vi "PicoScopeospaOpen.vi"(5 "Serial Number":string, 7 "Use Serial Number":bool, 8 "error in (no error)":errorcluster, 9 "Mode":u16(ring) items=["Dialog On Error", "no dialog - CloseUnit and Stop", "no dialog - Continue", "no dialog - Stop"], 10 "Resolution":u32(ring) items=["8-bit"=0, "12-bit"=1, "14-bit"=2, "15-bit"=3, "16-bit"=4, "10-bit"=10]) -> (0 "error out":errorcluster, 1 "Max ADC value":i16, 2 "Device Info":T2, 3 "handle out":i16, 4 "psospa Units":string, 6 "serialLth":i16)   [LabVIEW 2010]
doc: "This VI manages listing and opens devices with device details."
uses:
  psospa.dll
panel:
  out "PICO_USB_POWER_DETAILS":T1 {"dataPort_"."currentRdo_" format="%x"; "powerport_"."currentPdo_" format="%x"; "powerport_"."currentRdo_" format="%x"}
  out "minValue":i16
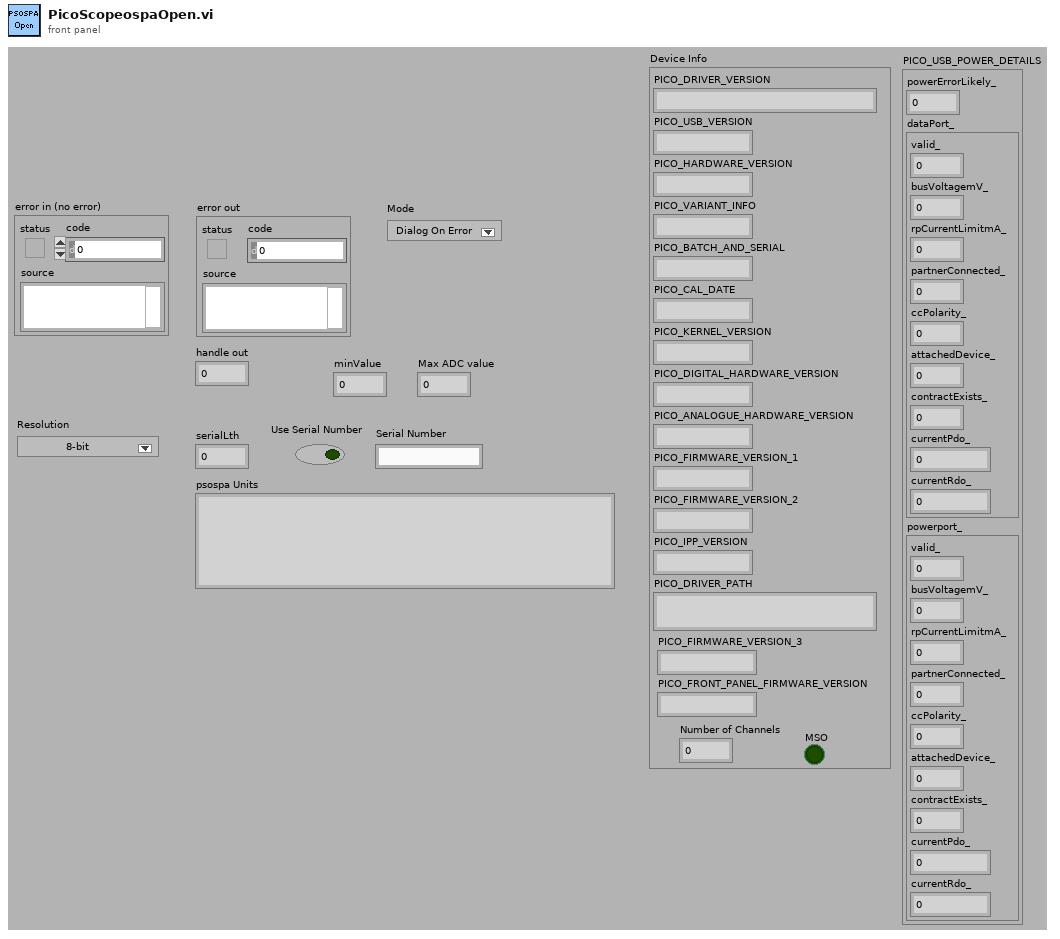
[diagram p1: front panel]
types:
  T1 = cluster{"powerErrorLikely_":u8, "dataPort_":cluster{"valid_":u8, "busVoltagemV_":u32, "rpCurrentLimitmA_":u32, "partnerConnected_":u8, "ccPolarity_":u8, "attachedDevice_":u32, "contractExists_":u8, "currentPdo_":u32, "currentRdo_":u32}, "powerport_":cluster{"valid_":u8, "busVoltagemV_":u32, "rpCurrentLimitmA_":u32, "partnerConnected_":u8, "ccPolarity_":u8, "attachedDevice_":u32, "contractExists_":u8, "currentPdo_":u32, "currentRdo_":u32}}
  T2 = cluster{"PICO_DRIVER_VERSION":string, "PICO_USB_VERSION":string, "PICO_HARDWARE_VERSION":string, "PICO_VARIANT_INFO":string, "PICO_BATCH_AND_SERIAL":string, "PICO_CAL_DATE":string, "PICO_KERNEL_VERSION":string, "PICO_DIGITAL_HARDWARE_VERSION":string, "PICO_ANALOGUE_HARDWARE_VERSION":string, "PICO_FIRMWARE_VERSION_1":string, "PICO_FIRMWARE_VERSION_2":string, "PICO_IPP_VERSION":string, "PICO_DRIVER_PATH":string, "PICO_FIRMWARE_VERSION_3":string, "PICO_FRONT_PANEL_FIRMWARE_VERSION":string, "Number of Channels":i16, "MSO":bool}
  T3 = cluster{"status":bool, "code":u32, "source":string}
  T4 = cluster{"PICO_DRIVER_VERSION":string, "PICO_USB_VERSION":string, "PICO_HARDWARE_VERSION":string, "PICO_VARIANT_INFO":string, "PICO_BATCH_AND_SERIAL":string, "PICO_CAL_DATE":string, "PICO_KERNEL_VERSION":string, "PICO_DIGITAL_HARDWARE_VERSION":string, "PICO_ANALOGUE_HARDWARE_VERSION":string, "PICO_FIRMWARE_VERSION_1":string, "PICO_FIRMWARE_VERSION_2":string, "PICO_IPP_VERSION":string, "PICO_DRIVER_PATH":string, "PICO_FIRMWARE_VERSION_3":string, "PICO_FRONT_PANEL_FIRMWARE_VERSION":string}
  T5 = cluster{"PICO_DRIVER_VERSION":string, "PICO_USB_VERSION":string, "PICO_HARDWARE_VERSION":string, "PICO_VARIANT_INFO":string, "PICO_BATCH_AND_SERIAL":string, "PICO_CAL_DATE":string, "PICO_KERNEL_VERSION":string, "PICO_DIGITAL_HARDWARE_VERSION":string, "PICO_ANALOGUE_HARDWARE_VERSION":string, "PICO_FIRMWARE_VERSION_1":string, "PICO_FIRMWARE_VERSION_2":string, "PICO_IPP_VERSION":string, "PICO_DRIVER_PATH":string, "PICO_FIRMWARE_VERSION_3":string, "PICO_FRONT_PANEL_FIRMWARE_VERSION":string, i16, bool}
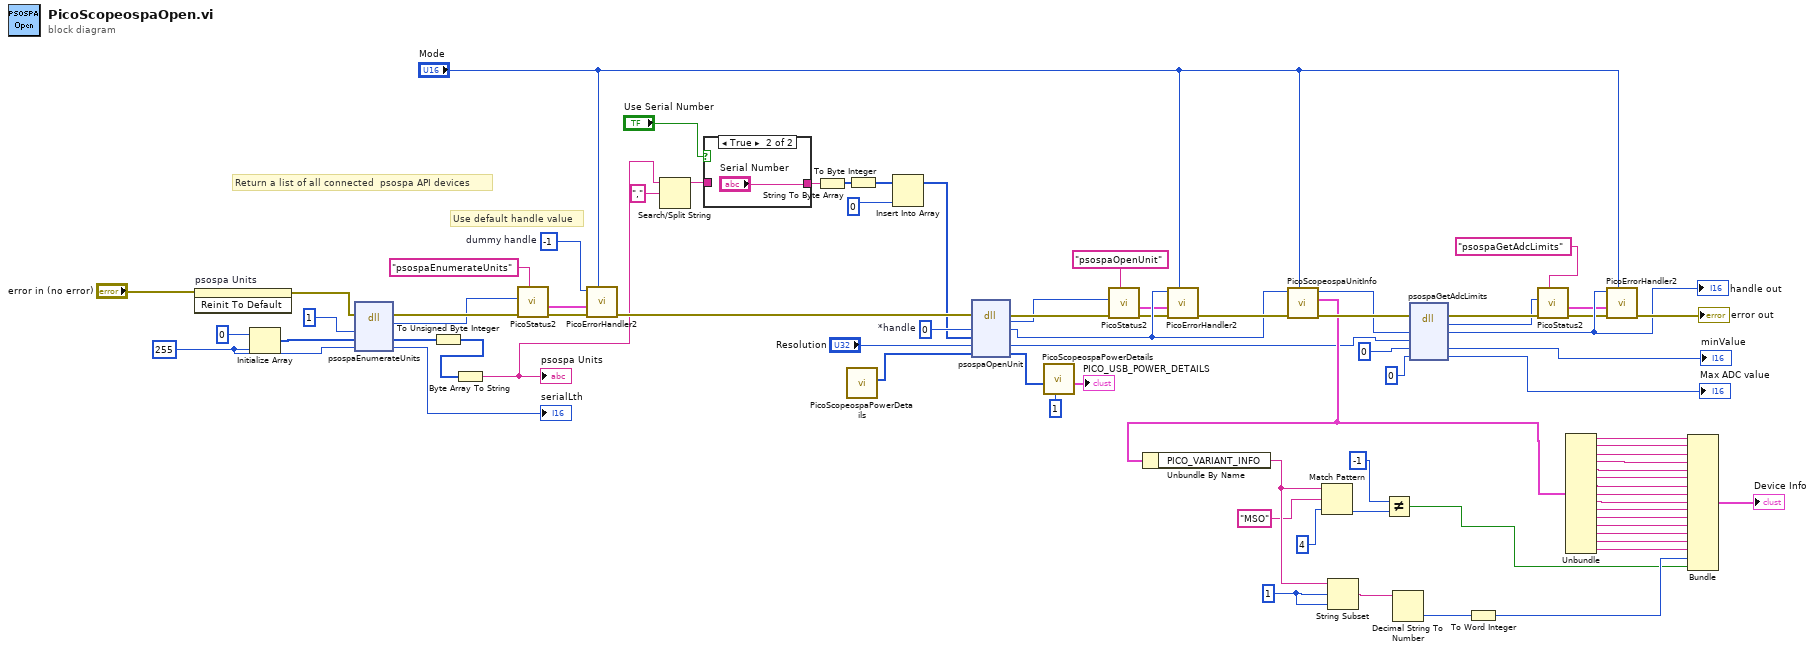
[diagram p0: block diagram]
diagram:
  w32 = i16 -1  # dummy handle
  w36 = i16 255 ("dimension size")
  w70 = 1 ("offset (0)")
  w44 = i16 0  # *handle
  # "Use default handle value"
  # "Return a list of all connected  psospa API devices"
  n1 = invoke on="psospa Units" class="Str" method="Reinit To Default"(error in="error in (no error)") -> (error out=w33:errorcluster)  [unwired: 2 in, 2 out]
  n2 = Initialize Array(i8 0 ("U8"), w36) -> (w38:i8[])
  n3 = dll-call lib="psospa.dll" fn="psospaEnumerateUnits"(error in=w33, "count"=i16 1, "serials"=w38, "serialLth"=w36) -> (error out=w28:errorcluster, "PICO_STATUS"=w27:u32, "serials"=w34:i8[], "serialLth"=→"serialLth":i16)  [unwired: 3 in, 1 out]
  n4 = To Unsigned Byte Integer(number=w34) -> (unsigned 8bit integer=w35:u8[])
  n5 = Byte Array To String(unsigned byte array=w35) -> (string=w18:string)
  "psospa Units" <- w18
  n6 = call "PicoStatus2.vi"("PICO source"="psospaEnumerateUnits" ("source"), "Error in"=w28, "PICO STATUS"=w27) -> ("error out"=w26:errorcluster, "PICO_STATUS out"=w25:T3)  [unwired: 5 in]
  n7 = call "PicoErrorHandler2.vi"("Mode"="Mode", "error in (no error)"=w26, "PICO_STATUS in"=w25, "handle In"=w32) -> ("error out"=w43:errorcluster)  [unwired: 7 in]
  n8 = Search/Split String(string=w18, search string/char (-)=",") -> (substring before match=w23:string)  [unwired: 1 in, 2 out]
  n9 = case shown="True" "Use Serial Number" {
    tunnel: w23 -> [w81 _]
    tunnel: [w81 "Serial Number"] -> w19
    frame False {
    }
    frame True {
    }
  }
  n10 = String To Byte Array(string=w19) -> (unsigned byte array=w21:u8[])
  n11 = call "PicoScopeospaPowerDetails.vi"() -> ("PICO_USB_POWER_DETAILS Out"=w1:u8[])  [unwired: 10 in, 1 out]
  n12 = To Byte Integer(number=w21) -> (8bit integer=w22:i8[])
  n13 = Insert Into Array(array=w22, new element=i8 0 ("new element/subarray")) -> (w16:i8[])  [unwired: 1 in]
  n14 = dll-call lib="psospa.dll" fn="psospaOpenUnit" ("ps3000.dll:_ps3000_open_unit@0")(error in=w43, "handle"=w44, "serial"=w16, "resolution"="Resolution", "powerDetails"=w1) -> (error out=w12:errorcluster, "PICO_STATUS"=w11:u32, "handle"=w31:i16, "resolution"=w41:u32, "powerDetails"=w3:u8[])  [unwired: 3 in, 1 out]
  n15 = call "PicoScopeospaPowerDetails.vi"("Function"=1, "PICO_USB_POWER_DETAILS In"=w3) -> ("PICO_USB_POWER_DETAILS"=→"PICO_USB_POWER_DETAILS":T1)  [unwired: 8 in, 1 out]
  n16 = call "PicoStatus2.vi"("PICO source"="psospaOpenUnit" ("source"), "Error in"=w12, "PICO STATUS"=w11) -> ("error out"=w15:errorcluster, "PICO_STATUS out"=w14:T3)  [unwired: 5 in]
  n17 = call "PicoErrorHandler2.vi"("Mode"="Mode", "error in (no error)"=w15, "PICO_STATUS in"=w14, "handle In"=w31) -> ("error out"=w80:errorcluster)  [unwired: 7 in]
  n18 = call "PicoScopeospaUnitInfo.vi"("Mode"="Mode", "error in (no error)"=w80, "handle in"=w31) -> ("error out"=w63:errorcluster, "Unit Info"=w56:T4, "handle out"=w61:i16)  [unwired: 6 in]
  n19 = Unbundle By Name(w56) -> ("PICO_VARIANT_INFO"=w69:string)
  n20 = Match Pattern(string=w69, regular expression="MSO", offset (0)=4) -> (offset past match=w66:i32)  [unwired: 3 out]
  n21 = String Subset(string=w69, offset (0)=w70, length (rest)=w70) -> (substring=w49:string)
  n22 = Not Equal?(x=-1, y=w66) -> (x != y?=w30:bool)
  n23 = Decimal String To Number(string=w49) -> (number=w46:i32)  [unwired: 2 in, 1 out]
  n24 = dll-call lib="psospa.dll" fn="psospaGetAdcLimits" ("ps3000.dll:_ps3000_open_unit@0")(error in=w63, "handle"=w61, "resolution"=w41, "minValue"=i16 0, "maxValue"=i16 0 ("manValue")) -> (error out=w7:errorcluster, "PICO_STATUS"=w6:u32, "handle"=w62:i16, "minValue"=→"minValue":i16, "maxValue"=→"Max ADC value":i16)  [unwired: 3 in, 1 out]
  "handle out" <- w62
  n25 = To Word Integer(number=w46) -> (16bit integer=w45:i16)
  n26 = call "PicoStatus2.vi"("PICO source"="psospaGetAdcLimits" ("source"), "Error in"=w7, "PICO STATUS"=w6) -> ("error out"=w10:errorcluster, "PICO_STATUS out"=w9:T3)  [unwired: 5 in]
  n27 = Unbundle(w56) -> ("PICO_DRIVER_VERSION"=w79:string, "PICO_USB_VERSION"=w78:string, "PICO_HARDWARE_VERSION"=w77:string, "PICO_VARIANT_INFO"=w76:string, "PICO_BATCH_AND_SERIAL"=w75:string, "PICO_CAL_DATE"=w74:string, "PICO_KERNEL_VERSION"=w73:string, "PICO_DIGITAL_HARDWARE_VERSION"=w72:string, "PICO_ANALOGUE_HARDWARE_VERSION"=w71:string, "PICO_FIRMWARE_VERSION_1"=w55:string, "PICO_FIRMWARE_VERSION_2"=w54:string, "PICO_IPP_VERSION"=w53:string, "PICO_DRIVER_PATH"=w52:string, "PICO_FIRMWARE_VERSION_3"=w51:string, "PICO_FRONT_PANEL_FIRMWARE_VERSION"=w50:string)
  n28 = call "PicoErrorHandler2.vi"("Mode"="Mode", "error in (no error)"=w10, "PICO_STATUS in"=w9, "handle In"=w62) -> ("error out"=→"error out":errorcluster)  [unwired: 7 in]
  n29 = Bundle("PICO_DRIVER_VERSION"=w79, "PICO_USB_VERSION"=w78, "PICO_HARDWARE_VERSION"=w77, "PICO_VARIANT_INFO"=w76, "PICO_BATCH_AND_SERIAL"=w75, "PICO_CAL_DATE"=w74, "PICO_KERNEL_VERSION"=w73, "PICO_DIGITAL_HARDWARE_VERSION"=w72, "PICO_ANALOGUE_HARDWARE_VERSION"=w71, "PICO_FIRMWARE_VERSION_1"=w55, "PICO_FIRMWARE_VERSION_2"=w54, "PICO_IPP_VERSION"=w53, "PICO_DRIVER_PATH"=w52, "PICO_FIRMWARE_VERSION_3"=w51, "PICO_FRONT_PANEL_FIRMWARE_VERSION"=w50, w45, w30) -> (→"Device Info":T5)  [unwired: 1 in]
